vi "Select Next Move.vi"(7 "Grove":T3[][](array[typedef]), 8 "Proposed Direction List":T4[](array[typedef]), 11 "Elf":T1[](array[typedef])) -> (3 "propose Moves":T2, 5 "Elf ID":i32)   [LabVIEW 2020]
uses:
  ENUM_Location Direction.ctl
  Cluster _Point Location.ctl
  RB ENUM_Spot ID.ctl
  MAP_Poroposed Moves.ctl
panel:
  out "Current Elf":T1
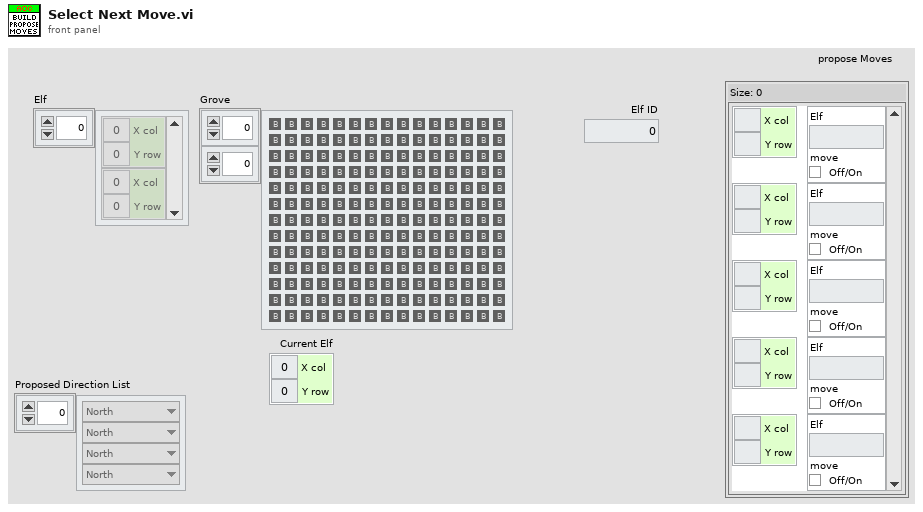
[diagram p1: front panel]
types:
  T1 = typedef "Cluster _Point Location.ctl" = cluster{"X col":i32, "Y row":i32}
  T2 = typedef "MAP_Poroposed Moves.ctl" = map{T1, cluster{"Elf":i32, "move":bool}}
  T3 = typedef "RB ENUM_Spot ID.ctl" = enum32{"Blank", "ELF", "Proposed"}
  T4 = typedef "ENUM_Location Direction.ctl" = enum16{"North", "North-East", "East", "South-East", "South", "South-West", "West", "North-West", "Center"}
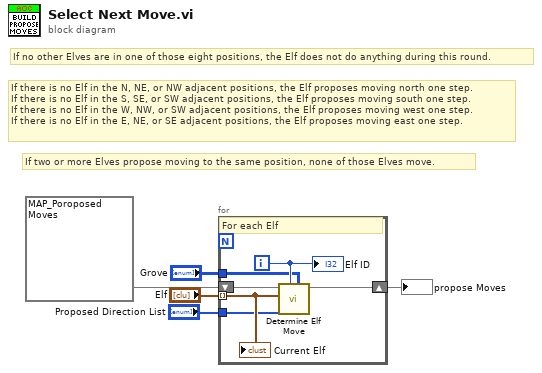
[diagram p0: block diagram]
diagram:
  # "If two or more Elves propose moving to the same position, none of those Elves move."
  # "If there is no Elf in the N, NE, or NW adjacent positions, the Elf proposes moving north one step.\nIf there is no Elf in the S, SE, or SW adjacent positions, the Elf proposes moving south one step.\nIf there is no Elf in the W, NW, or SW adjacent positions, the Elf proposes moving west one step.\nIf there is no Elf in the E, NE, or SE adjacent positions, the Elf proposes moving east one step."
  # "If no other Elves are in one of those eight positions, the Elf does not do anything during this round."
  n1 = for {
    tunnel: "Elf" -> [w9] mode=indexing
    tunnel: "Grove" -> [w7]
    shift-right: [w11] -> w1
    shift-left: T2 {} ("propose track") -> [w10]
    tunnel: "Proposed Direction List" -> [w6]
    i -> [w8]
    # "For each Elf"
    n2 = call "Determine Elf Move.vi"("Grove"=w7, "Eff ID"=w8, "Proposed Direction List"=w6, "Point"=w9, "Move Map"=w10) -> ("Move Map Out"=w11:T2)  [unwired: 6 in]
    "Current Elf" <- w9
    "Elf ID" <- w8
  }
  "propose Moves" <- w1
